vi "test_ResolveService_UpdateClusterId_ResolveServiceWorksWithoutError.vi"(8 "error in":errorcluster) -> (0 "error out":errorcluster, 2 "result":string, 3 "pass":bool)   [LabVIEW 2021, in "MeasurementServerTests.lvlib" / "Discovery Tests.lvlib"]
uses:
  Discovery Tests.lvlib
  gRPC/Generated APIs/ni/measurementlink/discovery/v1/RPC Messages/ni_measurementlink_discovery_v1_ResolveServiceRequest.ctl
  Runtime/Clients/Discovery V1/NI Discovery V1 Client.lvlib
  MeasurementServerTests.lvlib
  gRPC/Generated APIs/ni/measurementlink/discovery/v1/ni.measurementlink.discovery.v1.api.lvlib
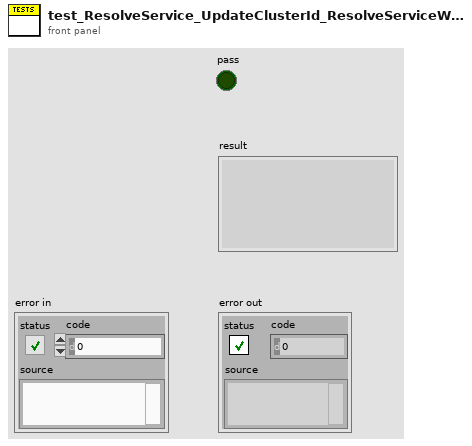
[diagram p1: front panel]
types:
  T1 = typedef "ni.measurementlink.discovery.v1.api.lvlib/ni_measurementlink_discovery_v1_ResolveServiceRequest.ctl" = cluster{"provided_interface":string, "service_class":string, "deployment_target":string, "version":string}
  T2 = typedef "ni.measurementlink.discovery.v1.api.lvlib/ni_measurementlink_discovery_v1_ServiceLocation.ctl" = cluster{"location":string, "insecure_port":string, "ssl_authenticated_port":string}
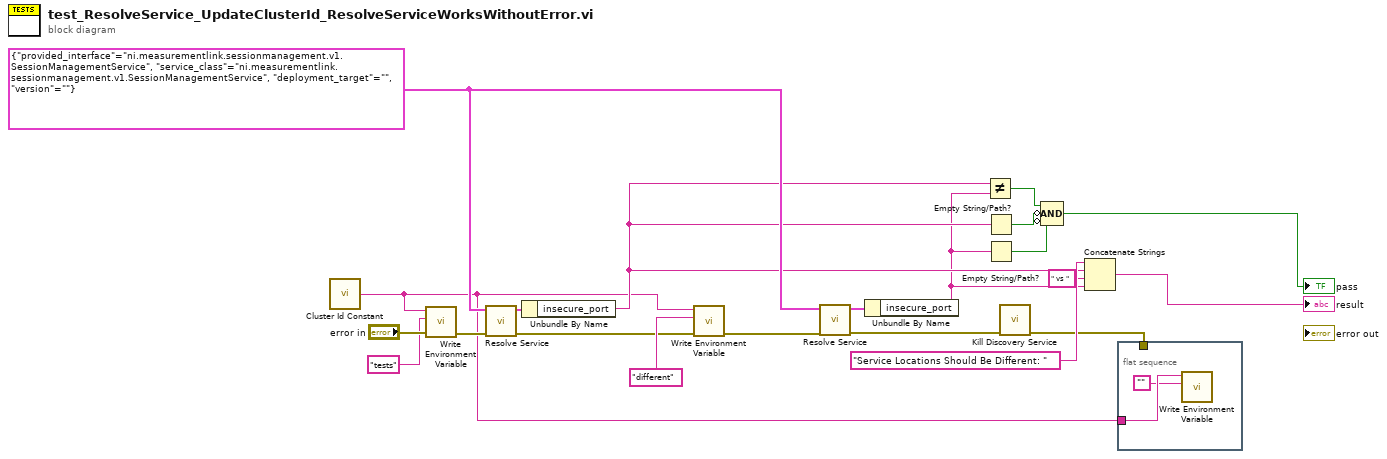
[diagram p0: block diagram]
diagram:
  w18 = T1 {"provided_interface"="ni.measurementlink.sessionmanagement.v1.SessionManagementService", "service_class"="ni.measurementlink.sessionmanagement.v1.SessionManagementService", "deployment_target"="", "version"=""} ("request data")
  n1 = call "Cluster Id Constant.vi"() -> ("cluster id env"=w1:string)
  n2 = call "Write Environment Variable.vi"("error in"="error in", "value"="tests", "name"=w1) -> ("error out"=w17:errorcluster)  [unwired: 8 in]
  n3 = call "Resolve Service.vi"("error in"=w17, "request data"=w18) -> ("error out"=w16:errorcluster, "response data"=w12:T2)  [unwired: 8 in]
  n4 = Unbundle By Name(w12) -> ("insecure_port"=w6:string)
  n5 = call "Write Environment Variable.vi"("error in"=w16, "value"="different", "name"=w1) -> ("error out"=w15:errorcluster)  [unwired: 8 in]
  n6 = call "Resolve Service.vi"("error in"=w15, "request data"=w18) -> ("error out"=w14:errorcluster, "response data"=w13:T2)  [unwired: 8 in]
  n7 = Unbundle By Name(w13) -> ("insecure_port"=w5:string)
  n8 = Not Equal?(x=w6, y=w5) -> (x != y?=w11:bool)
  n9 = Empty String/Path?(string/path=w6) -> (empty?=w10:bool)
  n10 = Empty String/Path?(string/path=w5) -> (empty?=w9:bool)
  n11 = call "Kill Discovery Service.vi"("error in"=w14) -> ("error out"=w2:errorcluster)  [unwired: 10 in]
  n12 = Compound Arithmetic op=AND(w11, invert w10, invert w9) -> (→"pass":bool)
  n13 = Concatenate Strings("Service Locations Should Be Different: " ("string"), w6, " vs " ("string"), w5) -> (→"result":string)
  n14 = flat-sequence {
    tunnel: w1 -> [w23]
    tunnel: w2 -> [_]
    frame #0 {
      n15 = call "Write Environment Variable.vi"("value"="", "name"=w23) -> ()  [unwired: 9 in, 1 out]
    }
  }
